vi "SerialINI.vi"(8 "error in (no error)":errorcluster caption="错误输入（无错误）", 10 "Serial INI":T1={"VISA串口名称"="COM20", "波特率"=9600, "数据位"=8, "奇偶校验"=enum."None", "停止位"=10, "流控制"=0, "超时"=10000, "终止符"=10, "启用终止符？"=FALSE} {"终止符" format="%.0x"; "流控制" items=["无", "XON/XOFF", "RTS/CTS", "XON/XOFF & RTS/CTS", "DTR/DSR", "XON/XOFF & DTR/DSR"]; "停止位" items=["1.0"=10, "1.5"=15, "2.0"=20]; "数据位" min=5 max=8 step=1}, 11 "serial 输入":refnum<class "serial.lvclass">) -> (0 "error out":errorcluster caption="错误输出", 3 "serial 输出":refnum<class "serial.lvclass">)   [LabVIEW 2019, in "serial.lvclass"]
uses:
  serial.lvclass
  serial.lvclass/serial.ctl
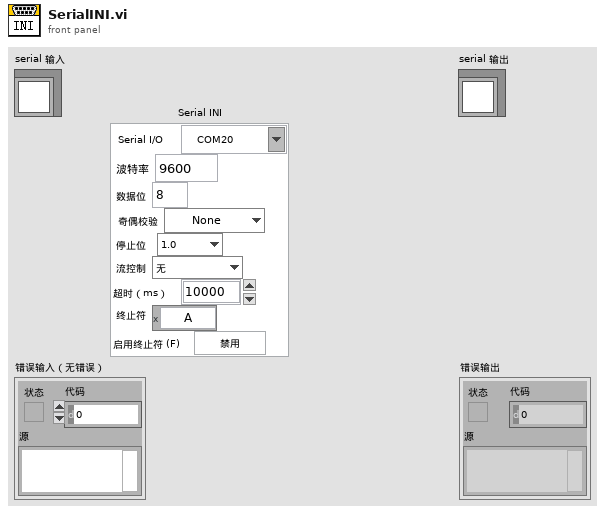
[diagram p1: front panel]
types:
  T1 = cluster{"VISA串口名称":refnum<visa-resource-name>, "波特率":u32, "数据位":u16, "奇偶校验":enum16{"None", "Odd", "Even", "Mark", "Space"}, "停止位":u16, "流控制":u16, "超时":u32, "终止符":u8, "启用终止符？":bool}
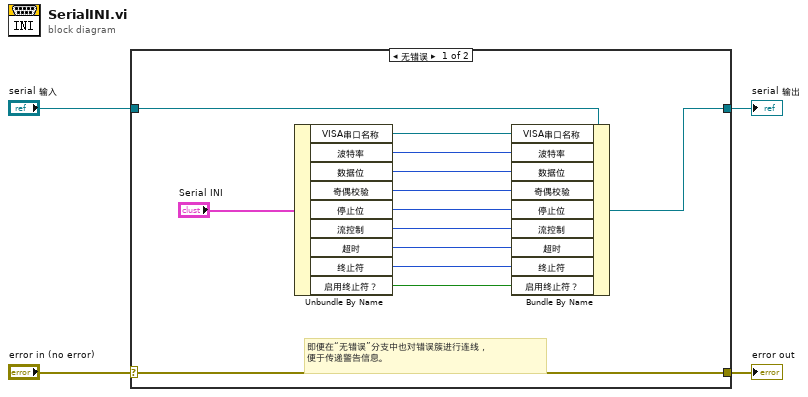
[diagram p0: block diagram]
diagram:
  n1 = case shown="无错误" "error in (no error)" {
    selector: "error in (no error)" -> [w17 w19]
    tunnel: [w17 w19] -> w3
    tunnel: [w5 w18] -> w1
    tunnel: "serial 输入" -> [w15 w18]
    frame No Error {
      # "即便在“无错误”分支中也对错误簇进行连线，\n便于传递警告信息。"
      n2 = Unbundle By Name("Serial INI") -> ("VISA串口名称"=w14:refnum<visa-resource-name>, "波特率"=w13:u32, "数据位"=w12:u16, "奇偶校验"=w11:enum16{"None", "Odd", "Even", "Mark", "Space"}, "停止位"=w10:u16, "流控制"=w9:u16, "超时"=w8:u32, "终止符"=w7:u8, "启用终止符？"=w6:bool)
      n3 = Bundle By Name(cluster=w15, "VISA串口名称"=w14, "波特率"=w13, "数据位"=w12, "奇偶校验"=w11, "停止位"=w10, "流控制"=w9, "超时"=w8, "终止符"=w7, "启用终止符？"=w6) -> (w5:refnum<class "serial.lvclass">)
    }
    frame Error {
    }
  }
  "error out" <- w3
  "serial 输出" <- w1
